vi "visuallyInspectPositionListResults3.vi"() -> ()   [LabVIEW 2016]
uses:
  <vilib>/vision/Image Controls.llb/IMAQ Image.ctl
  <vilib>/Utility/file.llb/Write Delimited Spreadsheet (DBL).vi
  <vilib>/regexp/Match Regular Expression.xnode
  <vilib>/vision/driver/NI_Vision_Acquisition_Software.lvlib
  <vilib>/vision/NI_Vision_Development_Module.lvlib
panel:
  out "Template 4":T1
  in  "Template Folder 4":path=path "C:/Users/Aerotech/cernbox/TargetsTable/Template4.png"
  out "Template 3":T1
  in  "Template Folder 3":path=path "C:/Users/Aerotech/cernbox/TargetsTable/Template3.png"
  out "Template 2":T1
  in  "Template Folder 2":path=path "C:/Users/Aerotech/cernbox/TargetsTable/Template2.png"
  in  "Tab Control":T2(tab)=enum."Camera Configurations"
  in  "Template Folder":path=path "C:/Users/Aerotech/cernbox/StabilityData/06_08SingleTarget/Template.png"
  in  "List of Interesting Locations":path=path "C:/Users/Aerotech/cernbox/StabilityData/06_08SingleTarget/Coordinates.csv"
  out "Pixel Y":dbl=1374.0
  out "Pixel X":dbl=1920.0
  in  "Nloops":i32=2000
  in  "Ncaptures":i32=1
  in  "File delimiter":string=","
  out "Number of Images":i32
  out "Template":T1
  in  "Camera gain":dbl(slide)=10.980988593155894 scale=0.0..16.0
  out "Thermometer [C]":dbl(slide)=nan scale=0.0..50.0
  in  "Coaxial light":bool=TRUE
  in  "Spotlights":bool=TRUE
  out "XYZ Stage Current Position":T3={"X [-750, 750 mm]"=-718.3709881209627, "Y [-150, 30 mm]"=141.8010543229765, "Z [-50, 50 mm]"=34.344995260000005}
  out "Finished!":bool=TRUE
  in  "Home?":bool
  in  "Axes Speeds [mm/s]":T4={"X Speed"=30.0, "Y Speed"=30.0, "Z Speed"=15.0}
  in  "Milliseconds to Wait":u32=5000
  in  "Camera Name":refnum<k21>="cam1" caption="IMAQdx Session"
  in  "Object Location [mm]":T5={"Go to X"=654.927, "Go to Y"=125.977, "Go to Z"=34.345}
  in  "Set of Coordinates to Process":dbl[][](array[numeric])
  in  "Settings":T6={"Algorithm"=2, "Number of Matches Requested"=1, "Minimum Match Score"=800.0, "SubPixel Accuracy"=TRUE, "Rotation Angle Ranges"=[], "Show Search Area"=FALSE, "Show Result"=TRUE} {"Rotation Angle Ranges"."End" format="%.1f"; "Rotation Angle Ranges"."Start" format="%.1f"; "Minimum Match Score" min=0 max=1000 format="%.2f"; "Number of Matches Requested" min=1; "Algorithm" items=["All", "Low Discrepancy Sampling", "Grayscale Value Pyramid", "Gradients Pyramid"]}
  out "Most recently collected image":T1(plugin-control)
  out "Image #":i32=2
  in  "error in (no error)":errorcluster
  out "Error report":errorcluster={"status"=TRUE, "code"=1172, "source"="Constructor Node Error creating instance of ControllerProperties in assembly Aerotech.A3200.LabVIEW.ControllerProperties, Aerotech.A3200.LabVIEW, Version=5.5.0.19, Culture=neutral, PublicKeyToken=478e72719c32735e, (System.NullReferenceException: Object reference not set to an instance of an object.) <append><b>System.NullReferenceException</b> in DisableMultiple.vi->visuallyInspectPositionListResults3.vi"}
  out "VISA error out":errorcluster={"status"=TRUE, "code"=7, "source"="Open File+.vi:Open File"}
  # "This VI can take pictures save the coordinates \nIt can also do the pattern matching at fly\nDifferent pattern could be matched but the template must be in the correct folder\nThe matched coordinates are in pixel which is to be later connverted into mm"
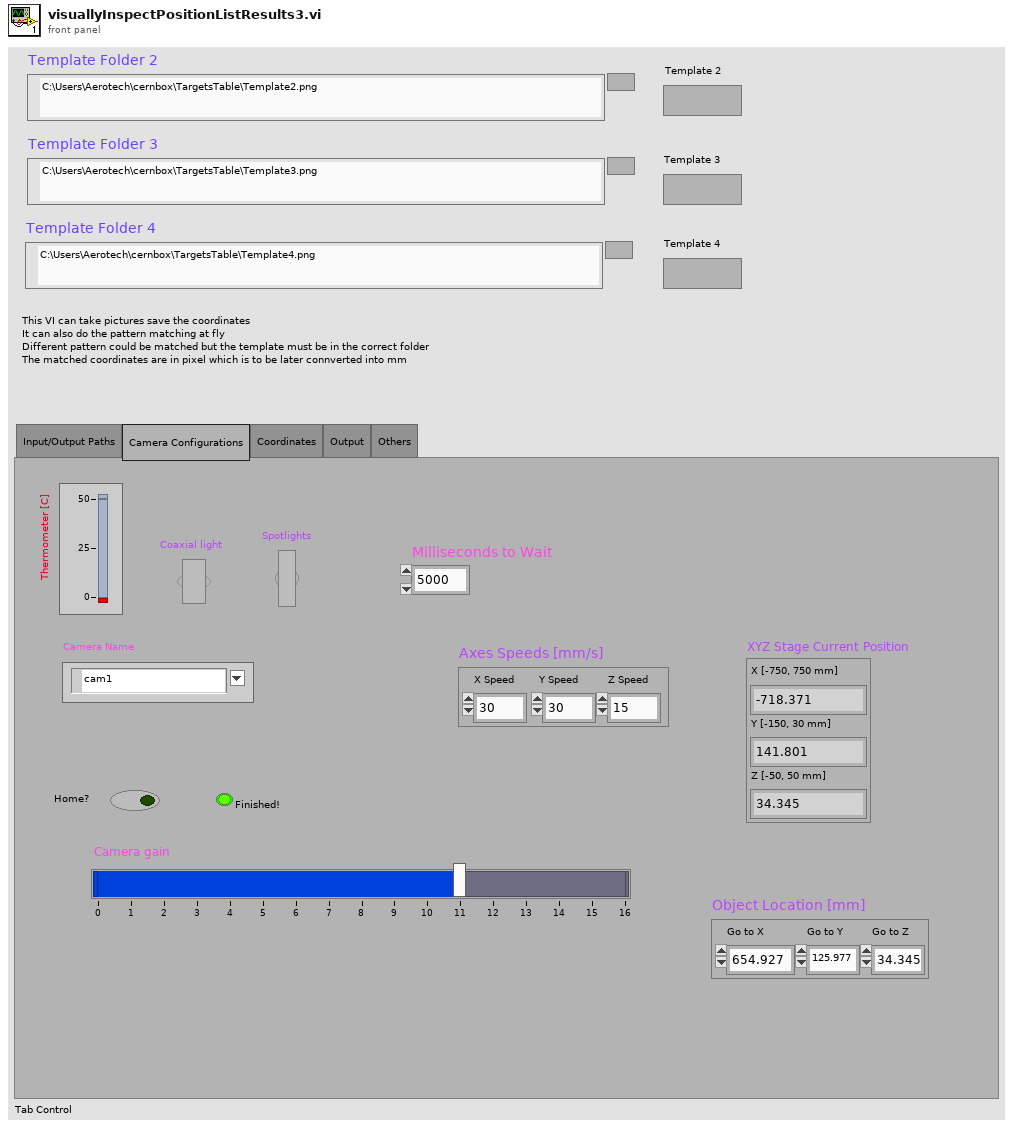
[diagram p1: front panel]
types:
  T1 = typedef "IMAQ Image.ctl" = refnum<image>
  T2 = enum32{"Input/Output Paths", "Camera Configurations", "Coordinates", "Output", "Others"}
  T3 = cluster{"X [-750, 750 mm]":dbl, "Y [-150, 30 mm]":dbl, "Z [-50, 50 mm]":dbl}
  T4 = cluster{"X Speed":dbl, "Y Speed":dbl, "Z Speed":dbl}
  T5 = cluster{"Go to X":dbl, "Go to Y":dbl, "Go to Z":dbl}
  T6 = cluster{"Algorithm":i32, "Number of Matches Requested":i32, "Minimum Match Score":sgl, "SubPixel Accuracy":bool, "Rotation Angle Ranges":cluster{"Start":sgl, "End":sgl}[], "Show Search Area":bool, "Show Result":bool}
  T7 = typedef "Image Type" = u32
  T8 = cluster{"Loaded array[0]":dbl, "Loaded array[1]":dbl, "Loaded array[2]":dbl, "Loaded array[3]":dbl, "Loaded array[4]":dbl, "Loaded array[5]":dbl, "Loaded array[6]":dbl, "Loaded array[7]":dbl, "Loaded array[8]":dbl}
  T9 = typedef "LabVIEW Interface for Arduino.lvlib/Arduino Resource.ctl" = cluster{"VISA resource":refnum<visa-resource-name>, "Board Type":T10, "Connection Type":enum8{"USB / Serial"}, "Bytes Per Packet (15)":u8}
  T10 = typedef "LabVIEW Interface for Arduino.lvlib/Board Type.ctl" = enum16{"Uno", "Dimuelanove w/Atmega 328", "Mega 2560"}
  T11 = typedef "ArduinoLT-ConfigurationControl.ctl" = cluster{"Lights: Digital I/O Pins":cluster{"Coaxial":u8, "Spotlights":u8}, "Thermistor Settings":cluster{"Analogue Readout Pin":u8, "Vcc Reference Pin":u8, "Paired Resistance (10K Ohms)":dbl, "Units (C)":enum16{"Celsius", "Fahrenheit", "Kelvin"}}}
  T12 = typedef "IMAQdx.ctl" = refnum<k21>
  T13 = cluster{"Set of Coordinates to Process[0]":dbl, "Set of Coordinates to Process[1]":dbl, "Set of Coordinates to Process[2]":dbl}
  T14 = cluster{"Final X":dbl, "Final Y":dbl, "Final Z":dbl}
  T15 = cluster{"Position":cluster{"x":sgl, "y":sgl}, "Angle":sgl, "Scale":sgl, "Score":sgl, "Bounding Box":cluster{"x":sgl, "y":sgl}[]}[]
  T16 = cluster{"Matches (pixel)[0]":cluster{"Position":cluster{"x":sgl, "y":sgl}, "Angle":sgl, "Scale":sgl, "Score":sgl, "Bounding Box":cluster{"x":sgl, "y":sgl}[]}, "Matches (pixel)[1]":cluster{"Position":cluster{"x":sgl, "y":sgl}, "Angle":sgl, "Scale":sgl, "Score":sgl, "Bounding Box":cluster{"x":sgl, "y":sgl}[]}, "Matches (pixel)[2]":cluster{"Position":cluster{"x":sgl, "y":sgl}, "Angle":sgl, "Scale":sgl, "Score":sgl, "Bounding Box":cluster{"x":sgl, "y":sgl}[]}, "Matches (pixel)[3]":cluster{"Position":cluster{"x":sgl, "y":sgl}, "Angle":sgl, "Scale":sgl, "Score":sgl, "Bounding Box":cluster{"x":sgl, "y":sgl}[]}, "Matches (pixel)[4]":cluster{"Position":cluster{"x":sgl, "y":sgl}, "Angle":sgl, "Scale":sgl, "Score":sgl, "Bounding Box":cluster{"x":sgl, "y":sgl}[]}, "Matches (pixel)[5]":cluster{"Position":cluster{"x":sgl, "y":sgl}, "Angle":sgl, "Scale":sgl, "Score":sgl, "Bounding Box":cluster{"x":sgl, "y":sgl}[]}, "Matches (pixel)[6]":cluster{"Position":cluster{"x":sgl, "y":sgl}, "Angle":sgl, "Scale":sgl, "Score":sgl, "Bounding Box":cluster{"x":sgl, "y":sgl}[]}, "Matches (pixel)[7]":cluster{"Position":cluster{"x":sgl, "y":sgl}, "Angle":sgl, "Scale":sgl, "Score":sgl, "Bounding Box":cluster{"x":sgl, "y":sgl}[]}, "Matches (pixel)[8]":cluster{"Position":cluster{"x":sgl, "y":sgl}, "Angle":sgl, "Scale":sgl, "Score":sgl, "Bounding Box":cluster{"x":sgl, "y":sgl}[]}}
  T17 = cluster{"Position":cluster{"x":sgl, "y":sgl}, "Angle":sgl, "Scale":sgl, "Score":sgl, "Bounding Box":cluster{"x":sgl, "y":sgl}[]}
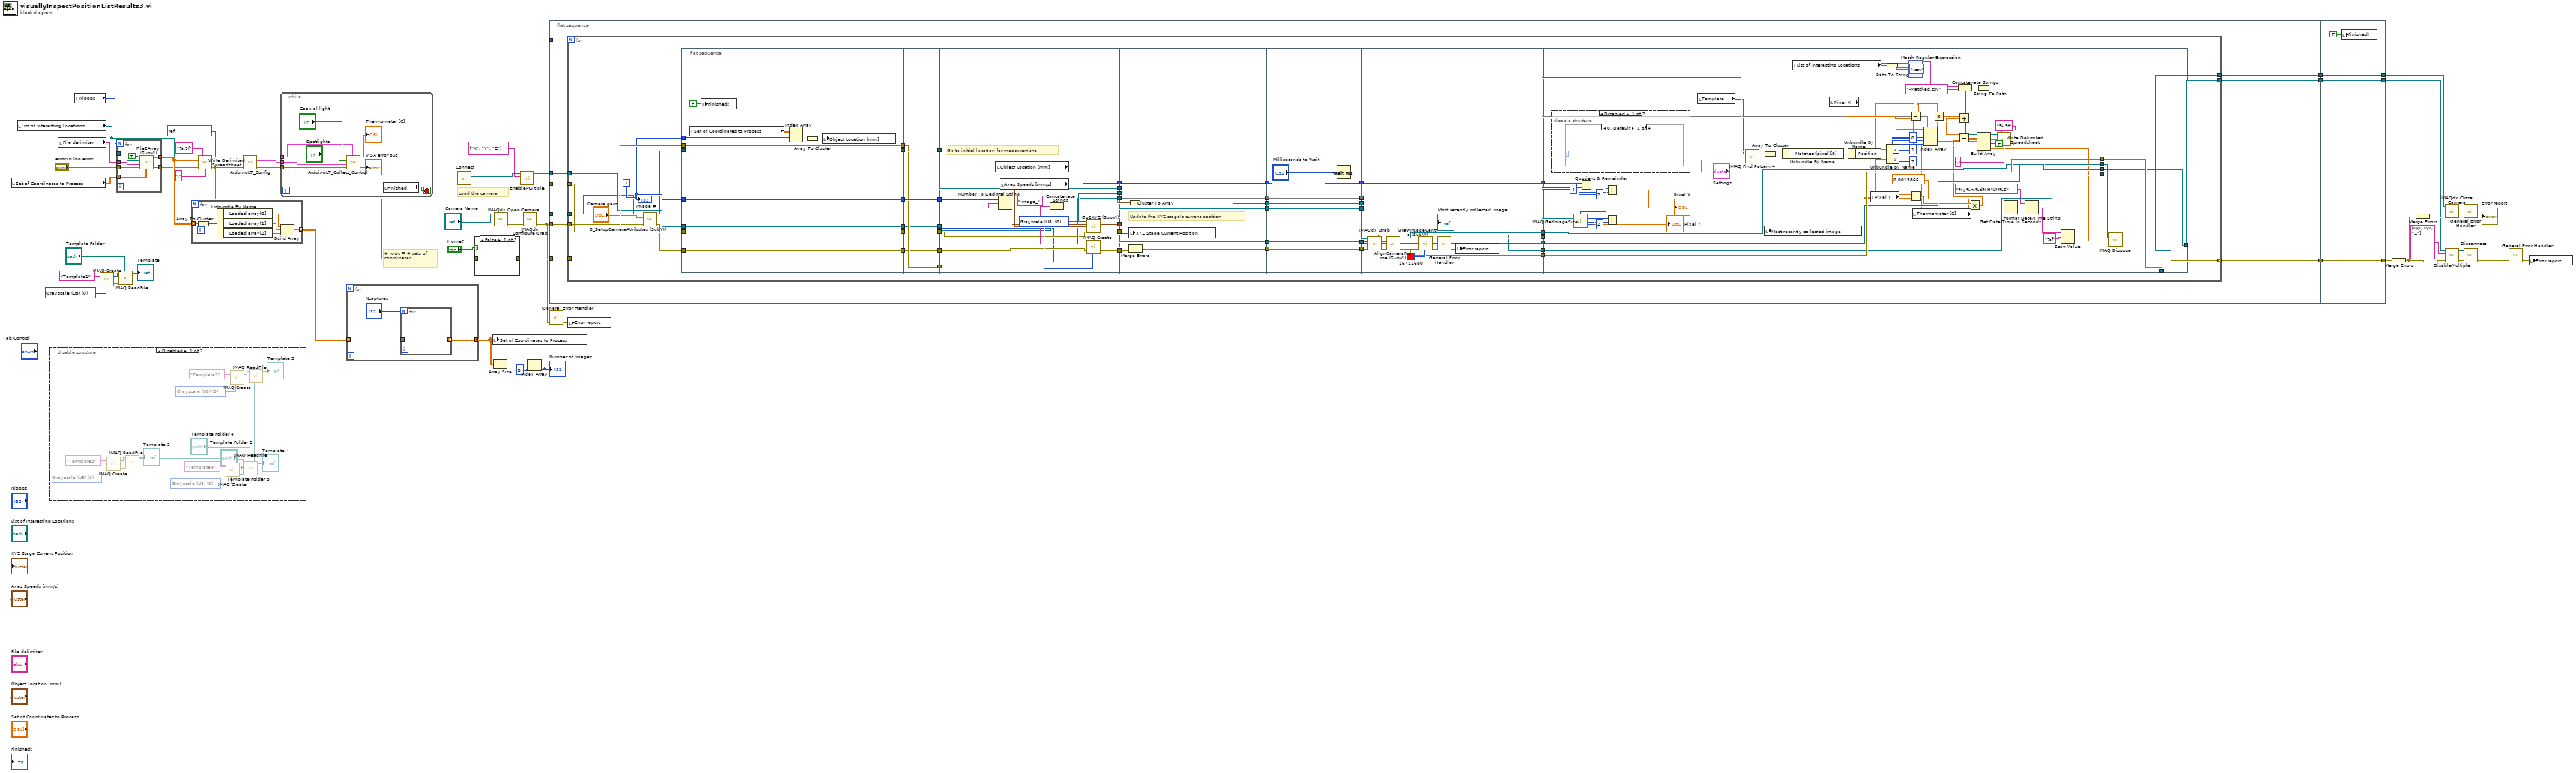
[diagram p0: block diagram]
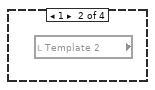
[diagram p3: hidden frame]
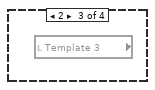
[diagram p4: hidden frame]
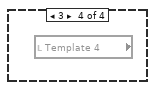
[diagram p5: hidden frame]
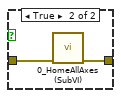
[diagram p7: hidden frame]
diagram:
  w10 = T7 0 items=["Grayscale (U8)", "Grayscale (I16)", "Grayscale (SGL)", "Complex (CSG)", "RGB (U32)", "HSL (U32)", "RGB (U64)", "Grayscale (U16)"] ("Image Type")
  # "# rows = # sets of\ncoordinates"
  # "Load the camera"
  n1 = local read "Set of Coordinates to Process"() -> (w44:dbl[][])
  n2 = local read "List of Interesting Locations"() -> (w43:path)
  n3 = disable-structure shown="Disabled" {
    frame Disabled {
      w58 = T7 0 items=["Grayscale (U8)", "Grayscale (I16)", "Grayscale (SGL)", "Complex (CSG)", "RGB (U32)", "HSL (U32)", "RGB (U64)", "Grayscale (U16)"] ("Image Type")
      w64 = T7 0 items=["Grayscale (U8)", "Grayscale (I16)", "Grayscale (SGL)", "Complex (CSG)", "RGB (U32)", "HSL (U32)", "RGB (U64)", "Grayscale (U16)"] ("Image Type")
      w70 = T7 0 items=["Grayscale (U8)", "Grayscale (I16)", "Grayscale (SGL)", "Complex (CSG)", "RGB (U32)", "HSL (U32)", "RGB (U64)", "Grayscale (U16)"] ("Image Type")
      n4 = call "IMAQ Create"("Image Name"="Template3", "Image Type"=w70) -> ("New Image"=w71:T1, "error out"=w69:errorcluster)  [unwired: 3 in]
      n5 = call "IMAQ ReadFile"("File Path"="Template Folder 2", "error in (no error)"=w69, "Image"=w71) -> ("Image Out"=→"Template 2":T1)  [unwired: 4 in, 4 out]
      n6 = call "IMAQ Create"("Image Name"="Template4", "Image Type"=w58) -> ("New Image"=w59:T1, "error out"=w57:errorcluster)  [unwired: 3 in]
      n7 = call "IMAQ Create"("Image Name"="Template2", "Image Type"=w64) -> ("New Image"=w65:T1, "error out"=w63:errorcluster)  [unwired: 3 in]
      n8 = call "IMAQ ReadFile"("File Path"="Template Folder 4", "error in (no error)"=w57, "Image"=w59) -> ("Image Out"=→"Template 4":T1)  [unwired: 4 in, 4 out]
      n9 = call "IMAQ ReadFile"("File Path"="Template Folder 3", "error in (no error)"=w63, "Image"=w65) -> ("Image Out"=→"Template 3":T1)  [unwired: 4 in, 4 out]
    }
    frame Enabled {
    }
  }
  n10 = local read "File delimiter"() -> (w46:string)
  n11 = local read "Nloops"() -> (w29:i32)
  n12 = call "IMAQ Create"("Image Name"="Template1", "Image Type"=w10) -> ("New Image"=w11:T1, "error out"=w9:errorcluster)  [unwired: 3 in]
  n13 = for {
    N: w29 -> [_]
    tunnel: w43 -> [w75]
    tunnel: w46 -> [w74]
    tunnel: w44 -> [w72]
    tunnel: [w78] -> w31 mode=concatenating
    tunnel: "error in (no error)" -> [w73]
    tunnel: [w77] -> w27
    n14 = call "File2Array (SubVI).vi"("Array for Processing"=w72, "error in (no error) in"=w73, "File delimiter"=w74, "Source array file"=w75, "Load array from file?"=TRUE) -> ("error in (no error) out"=w77:errorcluster, "Loaded array"=w78:dbl[][])  [unwired: 5 in]
  }
  n15 = call "IMAQ ReadFile"("File Path"="Template Folder", "error in (no error)"=w9, "Image"=w11) -> ("Image Out"=→"Template":T1)  [unwired: 4 in, 4 out]
  n16 = for {
    tunnel: w31 -> [w84] mode=indexing
    tunnel: [w80] -> w30 mode=indexing
    n17 = Array To Cluster(array=w84) -> (cluster=w83:T8)
    n18 = Unbundle By Name(w83) -> ("Loaded array[0]"=w82:dbl, "Loaded array[1]"=w81:dbl, "Loaded array[2]"=w79:dbl)
    n19 = Build Array(w82, w81, w79) -> (w80:dbl[])
  }
  n20 = call-poly <vilib>:"Write Delimited Spreadsheet.vi"("file path (dialog if empty)"=w43, "format (%.3f)"="%.9f", "2D data"=w31, "error in (no error)"=w27, "delimiter (\\t)"="," ("delimiter (\\t)")) -> ("error out"=w23:errorcluster)  [unwired: 9 in, 1 out]
  n21 = call "ArduinoLT_Config.vi"("error in"=w23, "VISA resource"=refnum<visa-resource-name> "LightsCTRL") -> ("error out"=w19:errorcluster, "Arduino Resource"=w22:T9, "Arduino Configuration OUT"=w21:T11)  [unwired: 3 in, 1 out]
  n22 = while {
    tunnel: w22 -> [w88]
    tunnel: w21 -> [w87]
    tunnel: w19 -> [w86]
    stop <- w89 stop-if-true
    n23 = call "ArduinoLT_Collect_Control.vi"("Arduino Configuration"=w87, "error in"=w86, "Arduino Resource IN"=w88, "Spotlights"="Spotlights", "Coaxial light"="Coaxial light") -> ("error out"=→"VISA error out":errorcluster, "Thermometer [C]"=→"Thermometer [C]":dbl)  [unwired: 4 in, 1 out]
    n24 = local read "Finished!"() -> (w89:bool)
  }
  n25 = for {
    tunnel: w30 -> [w94] mode=indexing
    tunnel: [w93] -> w15 mode=concatenating
    n26 = for {
      N: "Ncaptures" -> [_]
      tunnel: w94 -> [w96]
      tunnel: [w96] -> w93 mode=indexing
    }
  }
  n27 = call "Connect.vi"() -> ("error out"=w40:errorcluster, "controller"=w39:refnum<k24>)  [unwired: 10 in]
  n28 = case shown="False" "Home?" {
    tunnel: w23 -> [w97 w99]
    tunnel: [w97 w98] -> w50
    frame False {
    }
    frame True {
      n29 = call "0_HomeAllAxes (SubVI).vi"("error in (no error)"=w99) -> ("error out"=w98:errorcluster)  [unwired: 7 in, 3 out]
    }
  }
  n30 = local write "Set of Coordinates to Process"(w15) -> ()
  n31 = Array Size(array=w15) -> (size(s)=w17:i32[])
  n32 = call <vilib>:"IMAQdx Open Camera.vi"("Session In"="Camera Name") -> ("error out"=w52:errorcluster, "Session Out"=w53:T12)  [unwired: 2 in, 7 out]
  n33 = call "EnableMultiple.vi"("error in (no error)"=w40, "axis names"=string[] ["X", "Y", "Z"], "controller in"=w39) -> ("error out"=w37:errorcluster, "controller out"=w38:refnum<k24>)  [unwired: 7 in]
  n34 = call <vilib>:"IMAQdx Configure Grab.vi"("error in"=w52, "Session In"=w53) -> ("error out"=w24:errorcluster, "Session Out"=w25:T12)  [unwired: 8 out]
  n35 = Index Array(array=w17, index=0) -> (element=w16:i32)
  "Number of Images" <- w16
  n36 = flat-sequence {
    tunnel: w16 -> [w108]
    tunnel: w50 -> [w107]
    tunnel: w38 -> [w105]
    tunnel: w37 -> [w104]
    tunnel: w25 -> [w103]
    tunnel: w24 -> [w102]
    tunnel: [w106] -> w3
    tunnel: [w101] -> w2
    tunnel: [w100] -> w1
    tunnel: [w400] -> w4
    tunnel: [w401] -> w5
    tunnel: [w402] -> w49
    tunnel: w3 -> [w402]
    tunnel: w2 -> [w401]
    tunnel: w1 -> [w400]
    frame #0 {
      n37 = for {
        N: w108 -> [_]
        tunnel: w107 -> [w152]
        tunnel: [w148] -> w106 mode=indexing
        tunnel: w105 -> [w145]
        tunnel: w104 -> [w144]
        tunnel: w103 -> [w128]
        tunnel: w102 -> [w127]
        tunnel: [w120] -> w101
        tunnel: [w119] -> w100
        i -> [w129]
        n38 = call "0_SetupCameraAttributes (SubVI).vi"("error in (no error)"=w127, "Gain"="Camera gain", "Camera session in"=w128) -> ("error out"=w124:errorcluster, "Camera session out"=w126:T12)  [unwired: 7 in]
        n39 = flat-sequence {
          tunnel: w129 -> [w169]
          tunnel: w129 -> [w168]
          tunnel: [w168] -> w141
          tunnel: [w167] -> w139
          tunnel: w126 -> [w167]
          tunnel: [w166] -> w137
          tunnel: w152 -> [w166]
          tunnel: [w162] -> w135
          tunnel: w124 -> [w162]
          tunnel: [w164] -> w133
          tunnel: w145 -> [w164]
          tunnel: w144 -> [w163]
          tunnel: [w163] -> w131
          tunnel: w141 -> [w178]
          tunnel: [w178] -> w140
          tunnel: w139 -> [w177]
          tunnel: [w177] -> w138
          tunnel: w137 -> [w176]
          tunnel: [w176] -> w136
          tunnel: w135 -> [w175]
          tunnel: [w175] -> w134
          tunnel: w133 -> [w174]
          tunnel: [w174] -> w132
          tunnel: w131 -> [w173]
          tunnel: [w173] -> w130
          tunnel: [w191] -> w161
          tunnel: [w190] -> w160
          tunnel: [w189] -> w159
          tunnel: w140 -> [w179]
          tunnel: [w186] -> w156
          tunnel: [w185] -> w153
          tunnel: w138 -> [w185]
          tunnel: w136 -> [_]
          tunnel: w134 -> [w183]
          tunnel: [w182] -> w149
          tunnel: w132 -> [w181]
          tunnel: w130 -> [w180]
          tunnel: [w179] -> w109
          tunnel: w161 -> [w196]
          tunnel: w160 -> [w199]
          tunnel: w159 -> [w197]
          tunnel: [w203] -> w157
          tunnel: w156 -> [w203]
          tunnel: [w202] -> w154
          tunnel: w153 -> [w202]
          tunnel: [w200] -> w150
          tunnel: w149 -> [w201]
          tunnel: [w198] -> w147
          tunnel: [w196] -> w143
          tunnel: [w195] -> w110
          tunnel: w109 -> [w195]
          tunnel: [w209] -> w158
          tunnel: w157 -> [w209]
          tunnel: [w208] -> w155
          tunnel: w154 -> [w208]
          tunnel: [w207] -> w151
          tunnel: w150 -> [w207]
          tunnel: w147 -> [w206]
          tunnel: [w206] -> w146
          tunnel: w143 -> [w205]
          tunnel: [w205] -> w142
          tunnel: [w204] -> w111
          tunnel: w110 -> [w204]
          tunnel: w158 -> [w226]
          tunnel: w155 -> [w225]
          tunnel: w151 -> [w223]
          tunnel: w146 -> [w221]
          tunnel: [w216] -> w117
          tunnel: [w221] -> w116
          tunnel: [w215] -> w115
          tunnel: w142 -> [w213]
          tunnel: [w213] -> w114
          tunnel: [w212] -> w113
          tunnel: [w211] -> w112
          tunnel: w111 -> [w211]
          tunnel: w117 -> [w280]
          tunnel: [w280] -> w123
          tunnel: w116 -> [w251]
          tunnel: w115 -> [w278]
          tunnel: [w278] -> w122
          tunnel: w114 -> [w279]
          tunnel: [w279] -> w121
          tunnel: [w243] -> w118
          tunnel: w113 -> [w243]
          tunnel: w112 -> [w234]
          tunnel: [w398] -> w148
          tunnel: w123 -> [w398]
          tunnel: w122 -> [w397]
          tunnel: w121 -> [w396]
          tunnel: [w396] -> w120
          tunnel: [w395] -> w119
          tunnel: w118 -> [w395]
          frame #0 {
            n40 = local read "Set of Coordinates to Process"() -> (w170:dbl[][])
            n41 = local write "Finished!"(FALSE ("Finished!")) -> ()
            n42 = Index Array(array=w170, index (row)=w169) -> (element=w171:dbl[])  [unwired: 1 in]
            n43 = Array To Cluster(array=w171) -> (cluster=w172:T13)
            n44 = local write "Object Location [mm]"(w172) -> ()
          }
          frame #1 {
          }
          frame #2 {
            w194 = T7 0 items=["Grayscale (U8)", "Grayscale (I16)", "Grayscale (SGL)", "Complex (CSG)", "RGB (U32)", "HSL (U32)", "RGB (U64)", "Grayscale (U16)"] ("Image Type")
            # "Go to initial location for measurement"
            n45 = local read "Object Location [mm]"() -> (w192:T5)
            n46 = Number To Decimal String(number=w179) -> (decimal integer string=w184:string)  [unwired: 1 in]
            n47 = local read "Axes Speeds [mm/s]"() -> (w193:T4)
            n48 = Concatenate Strings("image_" ("Image Name"), w184) -> (w187:string)
            n49 = call "Go2XYZ (SubVI).vi"(".NET Refnum in"=w181, "Go to Coordinates"=w192, "Axis Speeds"=w193, "error in (no error)"=w180) -> (".NET Refnum out"=w191:refnum<k24>, "Final Position"=w190:T14, "error out"=w189:errorcluster)  [unwired: 7 in, 2 out]
            n50 = call "IMAQ Create"("Image Name"=w187, "Image Type"=w194, "error in (no error)"=w183) -> ("New Image"=w186:T1, "error out"=w182:errorcluster)  [unwired: 1 in, 1 out]
          }
          frame #3 {
            # "Update the XYZ stage's current position"
            n51 = Cluster To Array(cluster=w199) -> (array=w198:dbl[])
            n52 = local write "XYZ Stage Current Position"(w199) -> ()
            n53 = Merge Errors(w197, w201) -> (w200:errorcluster)
          }
          frame #4 {
            n54 = Wait (ms)(milliseconds to wait="Milliseconds to Wait") -> ()  [unwired: 1 out]
          }
          frame #5 {
            n55 = call <vilib>:"IMAQdx Grab.vi"("error in"=w223, "Image In"=w226, "Session In"=w225) -> ("error out"=w222:errorcluster, "Image Out"=w224:T1, "Session Out"=w217:T12)  [unwired: 1 in, 5 out]
            n56 = call "AlignCameraFrame (SubVI).vi"("error in (no error)"=w222, "Image Src"=w224, "Camera session in"=w217) -> ("error out"=w219:errorcluster, "Image Dst Out"=w220:T1, "Camera session out"=w212:T12)  [unwired: 6 in]
            n57 = call "DrawImageCentre (SubVI).vi"("Axis colour"=u32 16711680, "error in (no error)"=w219, "Refnum in"=w220) -> ("error out"=w216:errorcluster, "Refnum out"=w215:T1)  [unwired: 7 in]
            "Most recently collected image" <- w215
            n58 = call <vilib>:"General Error Handler.vi"("error in (no error)"=w216) -> ("error out"=w214:errorcluster)  [unwired: 2 in, 12 out]
            n59 = local write "Error report"(w214) -> ()
          }
          frame #6 {
            w239 = 0.0015866 ("y")
            n60 = disable-structure shown="Disabled" {
              frame Disabled {
                n61 = case shown="0, Default" {
                  selector: _ -> [_ _ _ _]
                  frame 0, Default {
                  }
                  frame 1 {
                    n62 = local read "Template 2"() -> ()  [unwired: 1 out]
                  }
                  frame 2 {
                    n63 = local read "Template 3"() -> ()  [unwired: 1 out]
                  }
                  frame 3 {
                    n64 = local read "Template 4"() -> ()  [unwired: 1 out]
                  }
                }
              }
              frame Enabled {
              }
            }
            n65 = call "IMAQ GetImageSize"("Image"=w278) -> ("Y Resolution"=w252:i32, "X Resolution"=w277:i32)  [unwired: 3 in, 1 out]
            n66 = Quotient & Remainder(x=w234, y=4) -> ()  [unwired: 2 out]
            n67 = Divide(x=w277, y=2) -> (x/y=→"Pixel X":dbl)
            n68 = Divide(x=w252, y=2) -> (x/y=→"Pixel Y":dbl)
            n69 = local read "Template"() -> (w227:T1)
            n70 = call "IMAQ Find Pattern 4"("Image"=w278, "Template"=w227, "Settings"="Settings") -> ("Image Out"=w274:T1, "Matches (pixel)"=w273:T15)  [unwired: 6 in, 5 out]
            n71 = Array To Cluster(array=w273) -> (cluster=w272:T16)
            n72 = local write "Most recently collected image"(w274) -> ()
            n73 = Unbundle By Name(w272) -> ("Matches (pixel)[0]"=w271:T17)
            n74 = local read "List of Interesting Locations"() -> (w260:path)
            n75 = local read "Pixel X"() -> (w269:dbl)
            n76 = Unbundle By Name(w271) -> ("Position"=w270:cluster{"x":sgl, "y":sgl})
            n77 = local read "Pixel Y"() -> (w267:dbl)
            n78 = Path To String(path=w260) -> (string=w261:string)
            n79 = Unbundle By Name(w270) -> ("x"=w237:sgl, "y"=w268:sgl)
            n80 = xnode "Match Regular Expression"("input string"=w261, "regular expression"=".csv") -> ("before match"=w264:string)  [unwired: 4 in, 4 out]
            n81 = Subtract(x=w237, y=w269) -> (x-y=w242:dbl)
            n82 = Subtract(x=w268, y=w267) -> (x-y=w240:dbl)
            n83 = local read "Thermometer [C]"() -> (w238:dbl)
            n84 = Index Array(array=w251, index #1=0 ("index"), index #2=1 ("index"), index #3=2 ("index")) -> (element #1=w246:dbl, element #2=w236:dbl, element #3=w247:dbl)
            n85 = Multiply(x=w242, y=w239) -> (x*y=w241:dbl)
            n86 = Add(x=w241, y=w246) -> (x+y=w245:dbl)
            n87 = Concatenate Strings(w264, "-Matched.csv" ("name or relative path")) -> (w265:string)
            n88 = Multiply(x=w240, y=w239) -> (x*y=w235:dbl)
            n89 = Subtract(x=w236, y=w235) -> (x-y=w244:dbl)
            n90 = String To Path(string=w265) -> (path=w266:path)
            n91 = Get Date/Time In Seconds() -> (seconds since 1Jan1904=w232:timestamp)
            n92 = Format Date/Time String(time format string (%c)="%y%m%d%H%M%S", seconds (now)=w232) -> (date/time string=w230:string)  [unwired: 1 in]
            n93 = Scan Value(string=w230, format string="%f") -> (value=w228:dbl)  [unwired: 1 in, 1 out]
            n94 = Build Array(w245, w244, w247, w238, w228) -> (w257:dbl[])
            n95 = call-poly <vilib>:"Write Delimited Spreadsheet.vi"("file path (dialog if empty)"=w266, "format (%.3f)"="%.9f", "1D data"=w257, "append to file? (new file:F)"=TRUE, "delimiter (\\t)"="," ("delimiter (\\t)")) -> ()  [unwired: 9 in, 2 out]
          }
          frame #7 {
            n96 = call "IMAQ Dispose"("Image"=w397) -> ()  [unwired: 5 in, 1 out]
          }
        }
        "Image #" <- w129
      }
    }
    frame #1 {
      n97 = local write "Finished!"(TRUE) -> ()
    }
  }
  n98 = call <vilib>:"General Error Handler.vi"("error in (no error)"=w24) -> ("error out"=w48:errorcluster)  [unwired: 2 in, 12 out]
  n99 = local write "Error report"(w48) -> ()
  n100 = Merge Errors(w49) -> (w34:errorcluster)
  n101 = Merge Errors(w34) -> (w13:errorcluster)
  n102 = call <vilib>:"IMAQdx Close Camera.vi"("error in"=w13, "Session In"=w4) -> ("error out"=w12:errorcluster)  [unwired: 9 out]
  n103 = call "DisableMultiple.vi"("error in (no error)"=w34, "axis names"=string[] ["X", "Y", "Z"], "controller in"=w5) -> ("error out"=w33:errorcluster, "controller out"=w35:refnum<k24>)  [unwired: 7 in]
  n104 = call <vilib>:"General Error Handler.vi"("error in (no error)"=w12) -> ("error out"=→"Error report":errorcluster)  [unwired: 2 in, 12 out]
  n105 = call "Disconnect.vi"("error in (no error)"=w33, "controller"=w35) -> ("error out"=w36:errorcluster)  [unwired: 9 in]
  n106 = call <vilib>:"General Error Handler.vi"("error in (no error)"=w36) -> ("error out"=w42:errorcluster)  [unwired: 2 in, 12 out]
  n107 = local write "Error report"(w42) -> ()
